vi "Compute I-V Curve.vi"(8 "error in (no error)":errorcluster, 11 "Waveform":waveform(dbl)) -> (0 "error out":errorcluster, 2 "Merged Graph Data":T1)   [LabVIEW 2013, in "Diode Characterization.lvlib" / "Diode IV.lvclass"]
uses:
  Diode IV.lvclass
  graphdata.ctl
  <vilib>/Utility/miscctls.llb/LVAnnotationListTypeDef.ctl
  <vilib>/Utility/miscctls.llb/LVCursorListTypeDef.ctl
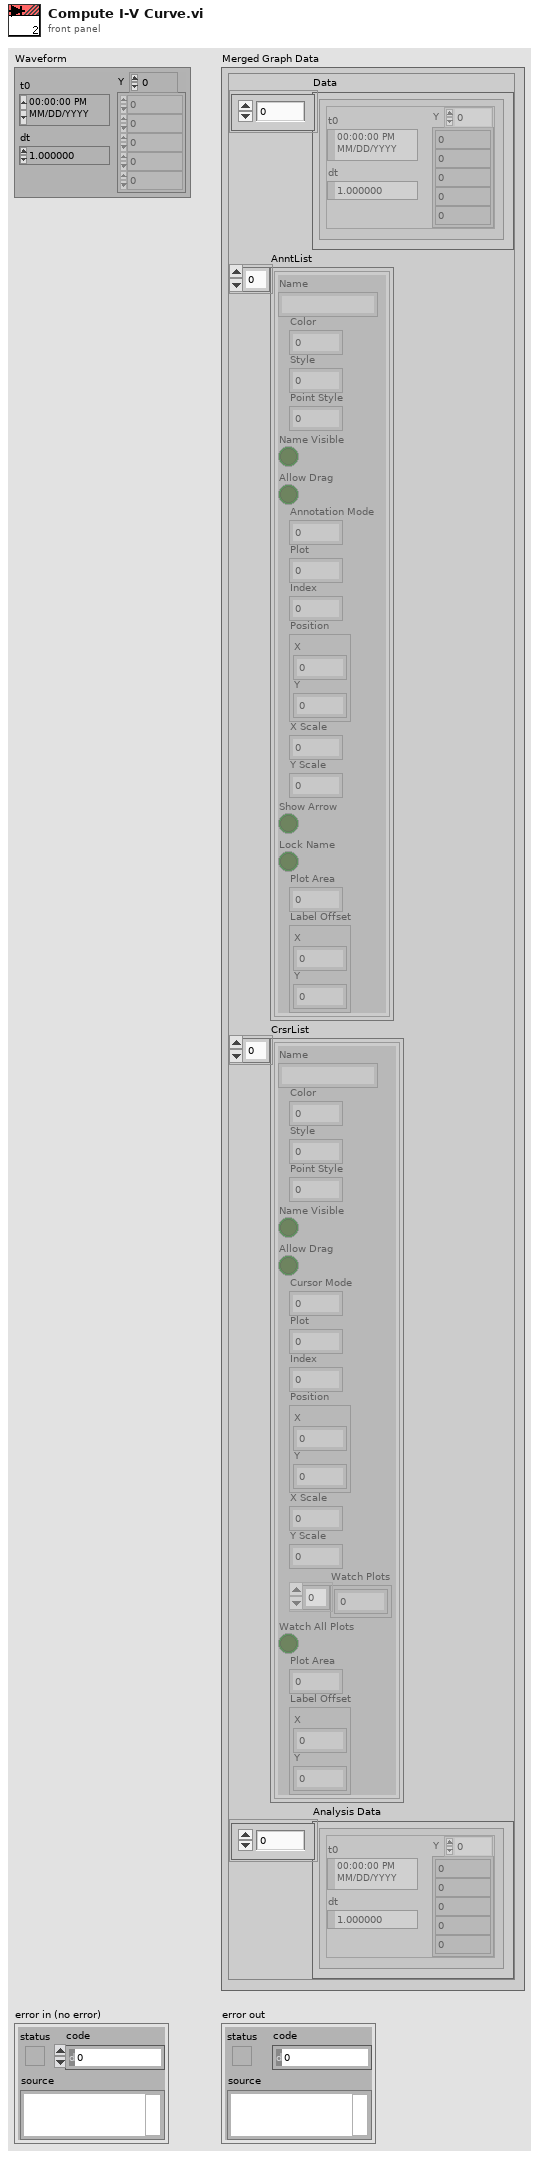
[diagram p1: front panel]
types:
  T1 = typedef "Diode Characterization.lvlib/Diode IV.lvclass/graphdata.ctl" = cluster{"Data":waveform(dbl)[], "AnntList":T2, "CrsrList":T3, "Analysis Data":waveform(dbl)[]}
  T2 = typedef "LVAnnotationListTypeDef.ctl" = cluster{"Name":string, "Color":u32, "Style":u8, "Point Style":u8, "Name Visible":bool, "Allow Drag":bool, "Annotation Mode":u32, "Plot":i32, "Index":i32, "Position":cluster{"X":dbl, "Y":dbl}, "X Scale":u32, "Y Scale":u32, "Show Arrow":bool, "Lock Name":bool, "Plot Area":i32, "Label Offset":cluster{"X":dbl, "Y":dbl}}[]
  T3 = typedef "LVCursorListTypeDef.ctl" = cluster{"Name":string, "Color":u32, "Style":u8, "Point Style":u8, "Name Visible":bool, "Allow Drag":bool, "Cursor Mode":u32, "Plot":i32, "Index":i32, "Position":cluster{"X":dbl, "Y":dbl}, "X Scale":u32, "Y Scale":u32, "Watch Plots":i32[], "Watch All Plots":bool, "Plot Area":i32, "Label Offset":cluster{"X":dbl, "Y":dbl}}[]
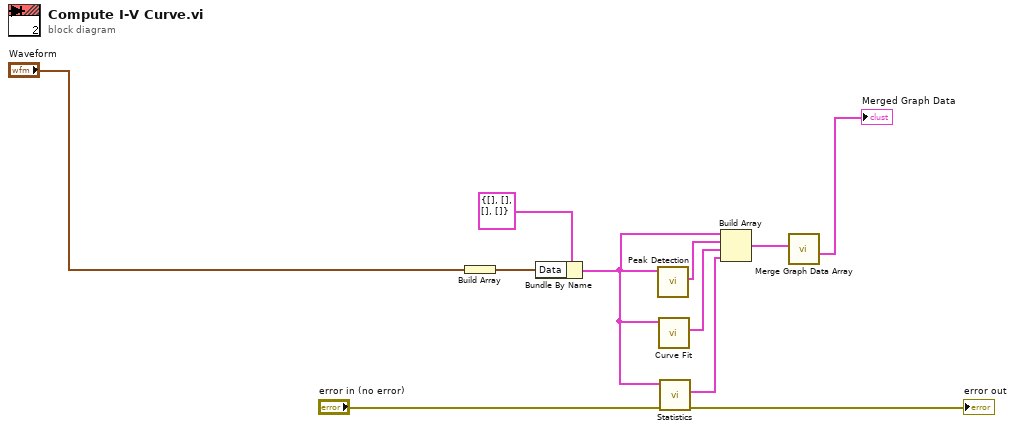
[diagram p0: block diagram]
diagram:
  n1 = Build Array("Waveform") -> (w2:waveform(dbl)[])
  n2 = Bundle By Name(cluster=T1 {"Data"=[], "AnntList"=[], "CrsrList"=[], "Analysis Data"=[]} ("Graph Data In"), "Data"=w2) -> (w8:T1)
  n3 = call "Peak Detection.vi"("Graph Data In"=w8) -> ("New Graph Data Out"=w4:T1)  [unwired: 8 in, 1 out]
  n4 = call "Curve Fit.vi"("Graph Data In"=w8) -> ("New Graph Data Out"=w6:T1)  [unwired: 8 in, 1 out]
  n5 = call "Statistics.vi"("error in (no error)"="error in (no error)", "Graph Data In"=w8) -> ("error out"=→"error out":errorcluster, "New Graph Data Out"=w7:T1)  [unwired: 7 in]
  n6 = Build Array(w8, w4, w6, w7) -> (w3:T1[])
  n7 = call "Merge Graph Data Array.vi"("Graph Data Array"=w3) -> ("Merged Graph Data"=→"Merged Graph Data":T1)  [unwired: 10 in]
